vi "Abort.vi"(8 "error in (no error)":errorcluster, 11 "Single Thread Test Runner In":refnum<class "Single Thread Test Runner.lvclass">) -> (0 "error out":errorcluster)   [LabVIEW 2020, in "Single Thread Test Runner.lvclass"]
uses:
  Single Thread Test Runner.lvclass
  Single Thread Test Runner.lvclass/Single Thread Test Runner.ctl
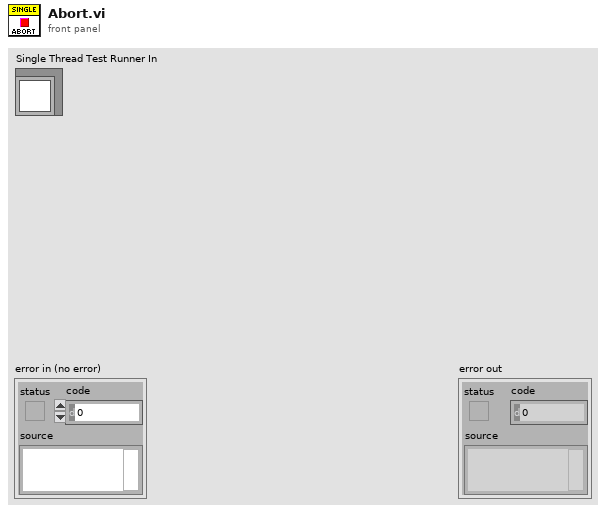
[diagram p1: front panel]
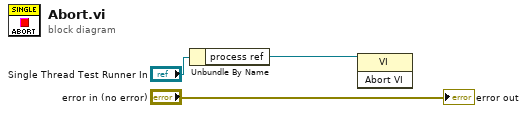
[diagram p0: block diagram]
diagram:
  n1 = Unbundle By Name("Single Thread Test Runner In") -> ("process ref"=w1:refnum<vi>)
  n2 = invoke class="VI" method="Abort VI"(reference=w1) -> ()  [unwired: 2 in, 3 out]
  "error out" <- "error in (no error)"
